vi "testInternalMemoryNew.vi"(8 "error in (no error)":errorcluster, 11 "TestCase in":refnum<class "Memory Manager Unit Tests.lvclass">) -> (0 "error out":errorcluster, 3 "TestCase out":refnum<class "Memory Manager Unit Tests.lvclass">)   [LabVIEW 2016, in "Memory Manager Unit Tests.lvclass"]
uses:
  Memory Manager Unit Tests.lvclass
  Library/Classes/Pointer/Memory.Pointer.lvclass/Memory.Pointer.ctl
  Library/Classes/Pointer/Accessors/Get Size.vi
  Library/Classes/Pointer/Accessors/Get Address.vi
  Library/Classes/Pointer/Accessors/Set Address.vi
  Library/Classes/Pointer/Accessors/Set Size.vi
  Library/Classes/Pointer.Internal/Memory.Pointer.Internal.lvclass
  C:/Git/Personal/LabVIEW-Memory-Manager/Source/Library/Classes/Pointer/Memory.Pointer.lvclass
  <vilib>/addons/_JKI Toolkits/VI Tester/TestCase.llb/TestCase.lvclass
  C:/Program Files (x86)/National Instruments/LabVIEW 2016/vi.lib/addons/_JKI Toolkits/VI Tester/TestCase.llb/TestCase.lvclass
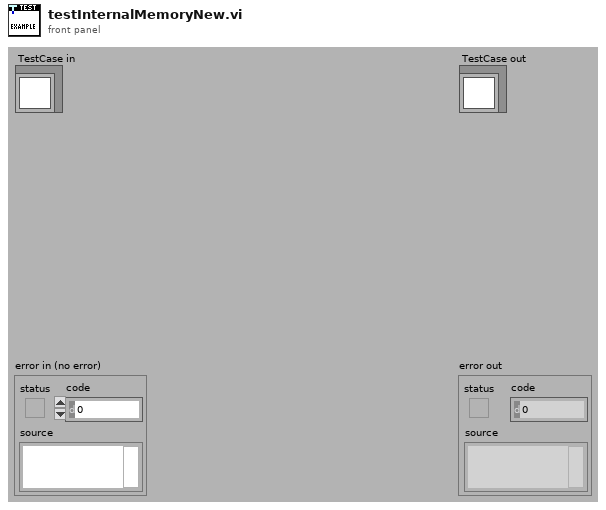
[diagram p1: front panel]
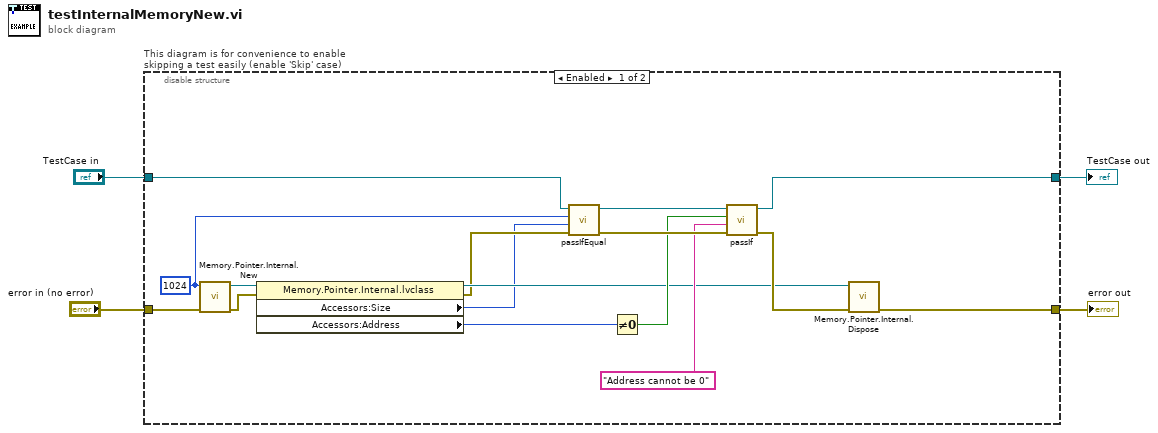
[diagram p0: block diagram]
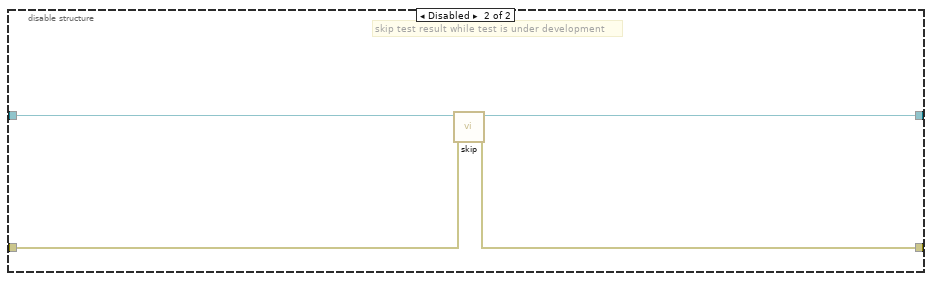
[diagram p2: hidden frame]
diagram:
  n1 = disable-structure "This diagram is for convenience to enable skipping a test easily (enable 'Skip' case)" shown="Enabled" {
    disable-tunnel: "TestCase in" -> [w20 w24]
    disable-tunnel: [w16 w22] -> w1
    disable-tunnel: [w18 w23] -> w3
    disable-tunnel: "error in (no error)" -> [w19 w21]
    frame Enabled {
      w5 = u64 1024 ("size")
      n2 = call "Memory.Pointer.Internal.New.vi"("error in (no error)"=w19, "size"=w5) -> ("error out"=w8:errorcluster, "pointer"=w10:refnum<class "Memory.Pointer.Internal.lvclass">)  [unwired: 8 in]
      n3 = property class="Memory.Pointer.Internal.lvclass"(reference=w10, error in=w8) -> (reference out=w9:refnum<class "Memory.Pointer.Internal.lvclass">, error out=w7:errorcluster, "Accessors:Size"=w6:u64, "Accessors:Address"=w13:u64)
      n4 = call-dynamic "passIfEqual.vi"("error in (no error)"=w7, "y"=w6, "x"=w5, "TestCase in"=w20) -> ("error out"=w15:errorcluster, "TestCase out"=w17:refnum<class "Memory Manager Unit Tests.lvclass">)  [unwired: 6 in]
      n5 = Not Equal To 0?(x=w13) -> (x != 0?=w12:bool)
      n6 = call-dynamic "passIf.vi"("error in (no error)"=w15, "message (\"\")"="Address cannot be 0" ("message (\"\")"), "pass"=w12, "TestCase in"=w17) -> ("error out"=w14:errorcluster, "TestCase out"=w16:refnum<class "Memory Manager Unit Tests.lvclass">)  [unwired: 6 in]
      n7 = call "Memory.Pointer.Internal.Dispose.vi"("error in (no error)"=w14, "pointer"=w9) -> ("error out"=w18:errorcluster)  [unwired: 9 in]
    }
    frame Disabled {
      # "skip test result while test is under development"
      n8 = call <vilib>:"skip.vi"("error in (no error)"=w21, "TestCase in"=w24) -> ("error out"=w23:errorcluster, "TestCase out"=w22:refnum<class "Memory Manager Unit Tests.lvclass">)  [unwired: 8 in]
    }
  }
  "error out" <- w3
  "TestCase out" <- w1
